vi "Display Unicode Strings in Table and List Box.vi"() -> ()   [LabVIEW 2009]
uses:
  _subVIs/tool_Unicode_Convert ASCII to Unicode (2D).vi
  _subVIs/tool_Unicode_Convert ASCII to Unicode (1D).vi
panel:
  in  "Headers":string[](array[string])=["Header 0", "Header 1", "Header 2"]
  in  "ASCII":string[][](array[string])=[["Option 00", "Option 01", "Option 02"], ["Option 10", "Option 11", "Option 12"], ["Option 20", "Option 21", "Option 22"]]
  out "Table Control":string[][](table)
  out "Multicolumn Listbox":i32(listbox)
  out "Listbox":i32(listbox)
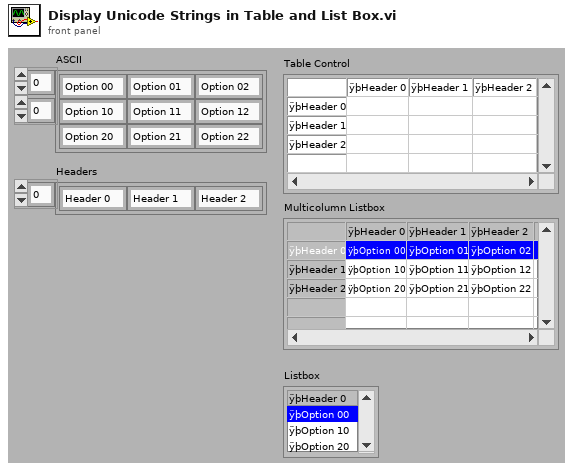
[diagram p1: front panel]
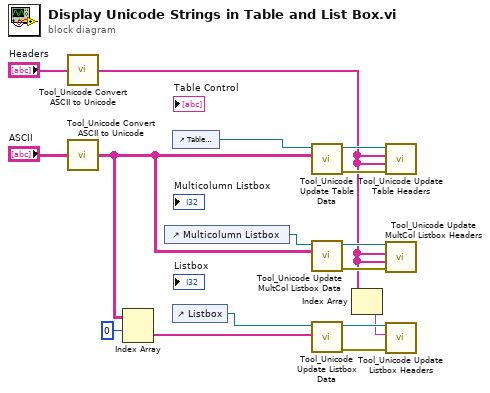
[diagram p0: block diagram]
diagram:
  n1 = call-poly "Tool_Unicode Convert ASCII to Unicode.vi"("ASCII"="Headers") -> ("Unicode"=w2:string[])  [unwired: 4 in]
  n2 = call-poly "Tool_Unicode Convert ASCII to Unicode.vi"("ASCII"="ASCII") -> ("Unicode"=w12:string[][])  [unwired: 4 in]
  n3 = Index Array(array=w12, index (row)=0) -> (element=w10:string[])  [unwired: 1 in]
  n4 = control-ref of="Multicolumn Listbox"() -> (w13:refnum<vi>)
  n5 = control-ref of="Table Control"() -> (w16:refnum<vi>)
  n6 = control-ref of="Listbox"() -> (w11:refnum<vi>)
  n7 = call "Tool_Unicode Update Table Data.vi"("Data[]"=w12, "Table Ref"=w16) -> ("error out"=w8:errorcluster, "Table Ref"=w9:refnum<vi>)  [unwired: 6 in]
  n8 = call "Tool_Unicode Update MultCol Listbox Data.vi"("Data[]"=w12, "Multicolumn Listbox Ref"=w13) -> ("error out"=w5:errorcluster, "Multicolumn Listbox Ref"=w6:refnum<vi>)  [unwired: 6 in]
  n9 = call "Tool_Unicode Update Listbox Data.vi"("Data[]"=w10, "Listbox Ref"=w11) -> ("error out"=w3:errorcluster, "Listbox Ref"=w4:refnum<vi>)  [unwired: 6 in]
  n10 = Index Array(array=w2) -> (element=w1:string)  [unwired: 1 in]
  n11 = call "Tool_Unicode Update Table Headers.vi"("error in (no error)"=w8, "Row Headers[]"=w2, "Column Headers[]"=w2, "Table Ref"=w9) -> ()  [unwired: 6 in, 2 out]
  n12 = call "Tool_Unicode Update MultCol Listbox Headers.vi"("error in (no error)"=w5, "Row Headers[]"=w2, "Column Headers[]"=w2, "Multicolumn Listbox Ref"=w6) -> ()  [unwired: 6 in, 2 out]
  n13 = call "Tool_Unicode Update Listbox Headers.vi"("error in (no error)"=w3, "Column Header"=w1, "Listbox Ref"=w4) -> ()  [unwired: 7 in, 2 out]
